vi "Flush Read.vi"(8 "error in (no error)":errorcluster, 11 "DeployResource in":refnum<class "DeployResource.lvclass">) -> (0 "error out":errorcluster, 2 "Data":string, 3 "DeployResource out":refnum<class "DeployResource.lvclass">)   [LabVIEW 2020]
uses:
  DeployResource.lvclass
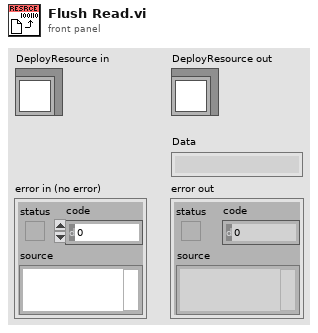
[diagram p1: front panel]
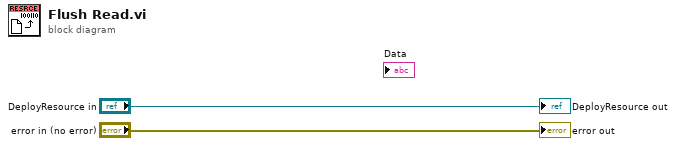
[diagram p0: block diagram]
diagram:
  "error out" <- "error in (no error)"
  "DeployResource out" <- "DeployResource in"
